vi "Andor_iXon_Point-mode.vi"(8 "Input Cluster 2":T6, 9 "Enum":enum32{"Picture", "Int Trace", "Video"}(ring), 10 "Cluster":T7) -> (0 "Output Cluster":T6, 1 "Numeric":dbl)   [LabVIEW 2009]
uses:
  atmcd32d.llb/AcquisitionMode_mode typedef.ctl
  atmcd32d.llb/ReadMode_mode typedef.ctl
  atmcd32d.llb/TriggerMode_mode typedef.ctl
  atmcd32d.llb/Shutter_type typedef.ctl
  atmcd32d.llb/Shutter_mode typedef.ctl
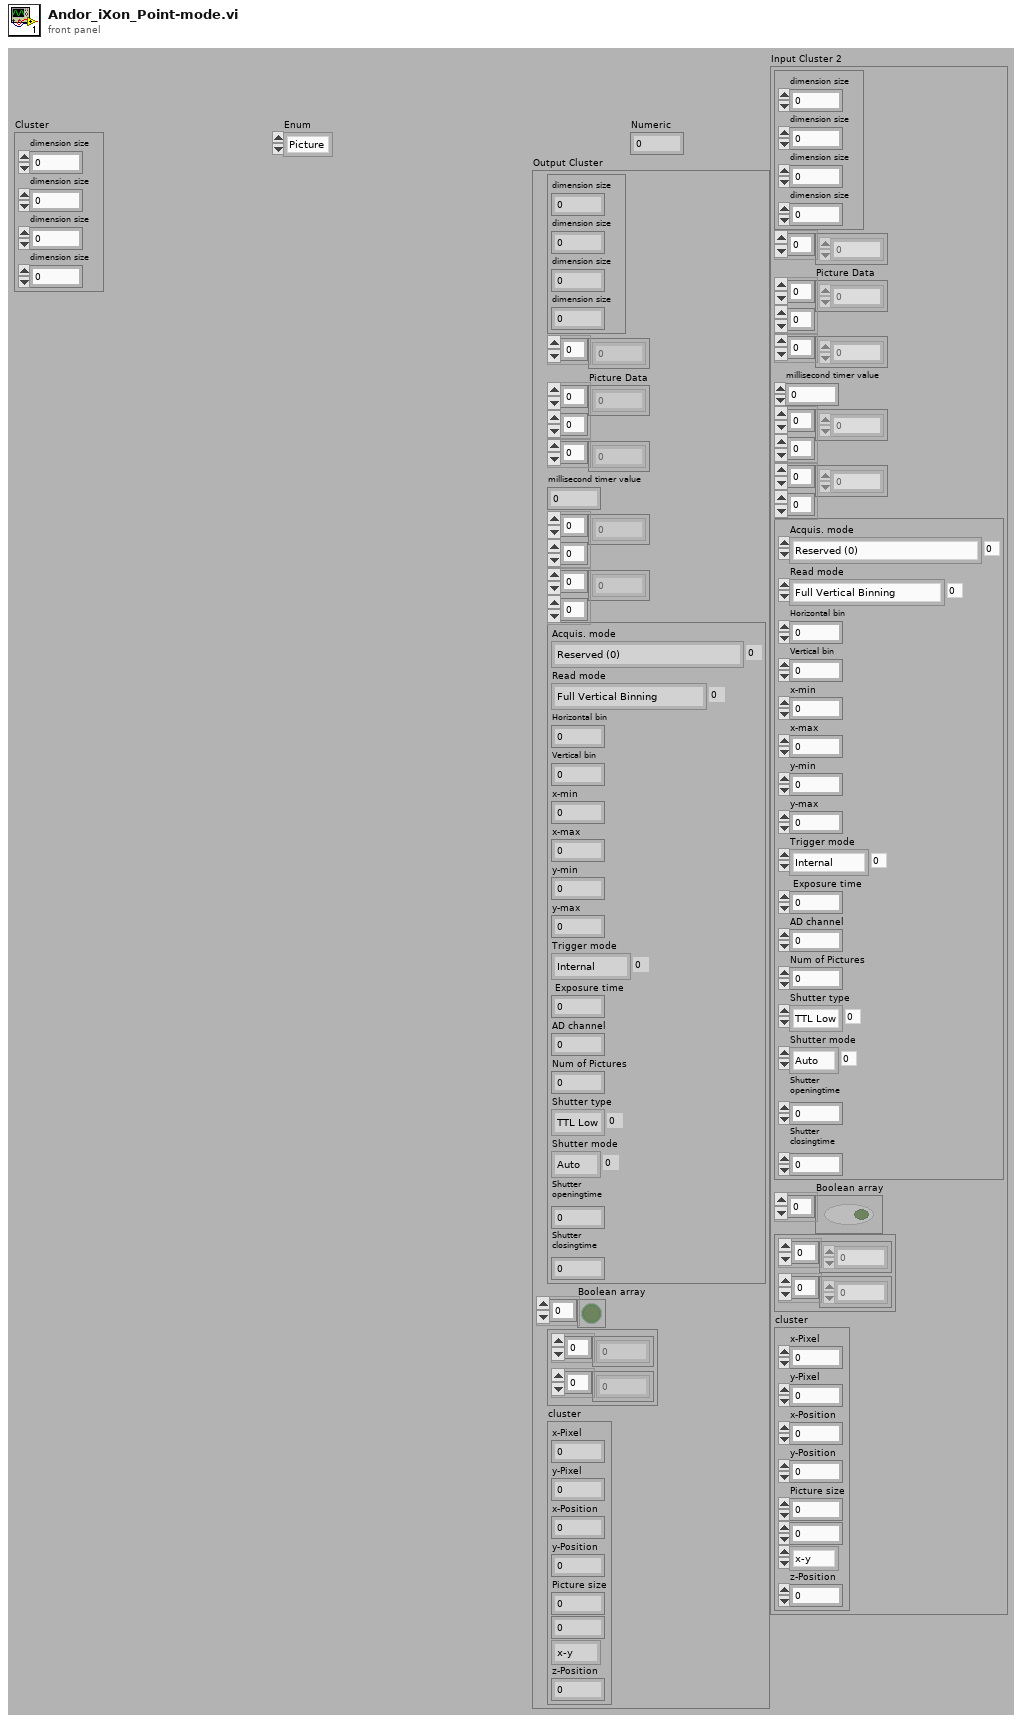
[diagram p1: front panel]
types:
  T1 = typedef "AcquisitionMode_mode typedef.ctl" = enum16{"Reserved (0)", "Single Scan", "Accumulate", "Kinetics", "Fast Kinetics", "Run Till Abort", "Reserved (6)", "Reserved (7)", "Reserved (8)", "Time Delayed Integration"}
  T2 = typedef "ReadMode_mode typedef.ctl" = enum16{"Full Vertical Binning", "Multi-Track", "Random-Track", "Single-Track", "Image"}
  T3 = typedef "TriggerMode_mode typedef.ctl" = enum16{"Internal", "External", "N/A (2)", "N/A (3)", "N/A (4)", "N/A (5)", "External Start"}
  T4 = typedef "Shutter_type typedef.ctl" = enum16{"TTL Low", "TTL High"}
  T5 = typedef "Shutter_mode typedef.ctl" = enum16{"Auto", "Open", "Close"}
  T6 = cluster{cluster{"dimension size":i32, "dimension size":i32, "dimension size":i32, "dimension size":i32}, i32[], "Picture Data":dbl[][], u32[], "millisecond timer value":u32, dbl[][], i32[][], cluster{"Acquis. mode":T1, "Read mode":T2, "Horizontal bin":i32, "Vertical bin":i32, "x-min":i32, "x-max":i32, "y-min":i32, "y-max":i32, "Trigger mode":T3, " Exposure time":sgl, "AD channel":i32, "Num of Pictures":i32, "Shutter type":T4, "Shutter mode":T5, "Shutter\nopeningtime":i32, "Shutter\nclosingtime":i32}, "Boolean array":bool[], cluster{dbl[], dbl[]}, "cluster":cluster{"x-Pixel":u16, "y-Pixel":u16, "x-Position":dbl, "y-Position":dbl, "Picture size":dbl, dbl, enum32{"x-y", "x-z", "y-z"}, "z-Position":dbl}}
  T7 = cluster{"dimension size":i32, "dimension size":i32, "dimension size":i32, "dimension size":i32}
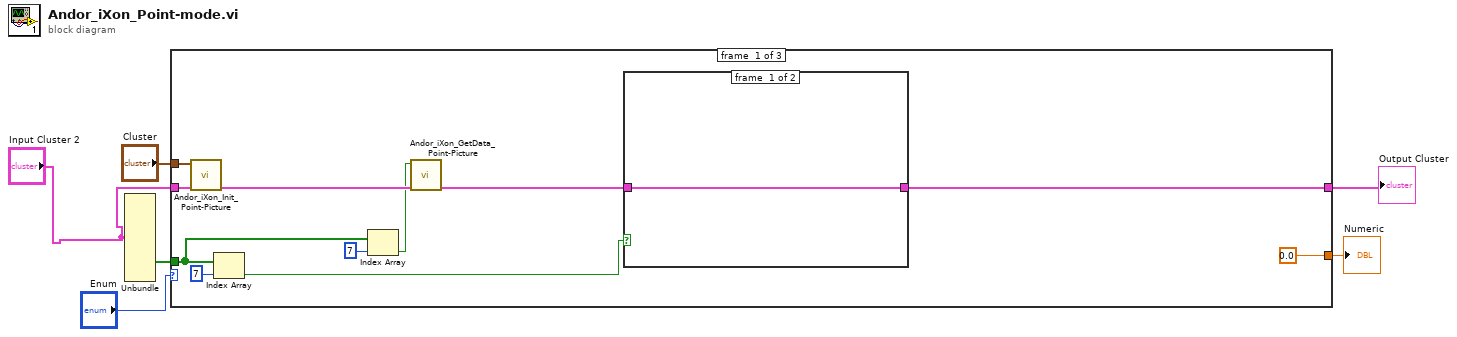
[diagram p0: block diagram]
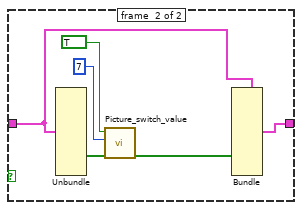
[diagram p2: hidden frame]
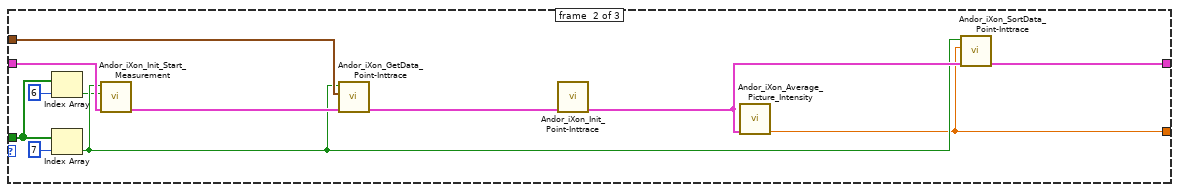
[diagram p3: hidden frame]
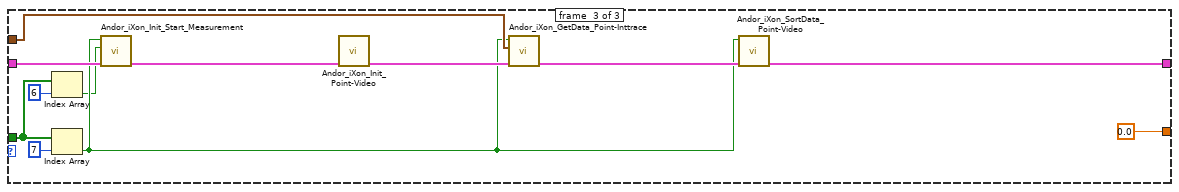
[diagram p4: hidden frame]
diagram:
  n1 = Unbundle("Input Cluster 2") -> ("Boolean array"=w3:bool[])  [unwired: 10 out]
  n2 = case shown="\"Video\"" "Enum" {
    tunnel: [w17 w32 w44] -> w2
    tunnel: "Cluster" -> [w13 w35 w47]
    tunnel: "Input Cluster 2" -> [w8 w31 w43]
    tunnel: w3 -> [w15 w27 w39]
    tunnel: [0.0 ("Numeric") w25 0.0 ("Numeric")] -> w5
    frame #0 {
      n3 = call "Andor_iXon_Init_Point-Picture.vi"("Input Cluster 2"=w8, "Cluster"=w13) -> ("Output Cluster"=w14:T6)  [unwired: 9 out]
      n4 = Index Array(array=w15, index=7) -> (element=w9:bool)
      n5 = Index Array(array=w15, index=7) -> (element=w11:bool)
      n6 = call "Andor_iXon_GetData_Point-Picture.vi"("Input Cluster"=w14, "Measure"=w11) -> ("Output Cluster"=w16:T6)  [unwired: 9 out]
      n7 = case shown="True" w9 {
        tunnel: w16 -> [w18 w21]
        tunnel: [w18 w19] -> w17
        frame #0 {
        }
        frame #1 {
          n8 = Unbundle(w21) -> ("Boolean array"=w22:bool[])  [unwired: 10 out]
          n9 = call "Picture_switch_value.vi"("Boolean array in"=w22, "Value to switch"=7, "Switch"=TRUE) -> ("Boolean array out"=w20:bool[])  [unwired: 8 out]
          n10 = Bundle(cluster=w21, "Boolean array"=w20) -> (w19:T6)  [unwired: 10 out]
        }
      }
    }
    frame #1 {
      n11 = Index Array(array=w27, index=6) -> (element=w26:bool)
      n12 = Index Array(array=w27, index=7) -> (element=w29:bool)
      n13 = call "Andor_iXon_Init_Start_Measurement.vi"("Input Cluster 2"=w31, "change"=w26, "Init"=w29) -> ("Input Cluster 3"=w30:T6)  [unwired: 8 out]
      n14 = call "Andor_iXon_GetData_Point-Inttrace.vi"("Input Cluster"=w30, "Cluster"=w35, "Measure"=w29) -> ("Output Cluster"=w34:T6)  [unwired: 8 out]
      n15 = call "Andor_iXon_Init_Point-Inttrace.vi"("Input Cluster"=w34) -> ("Input Cluster 2"=w33:T6)  [unwired: 10 out]
      n16 = call "Andor_iXon_Average_Picture_Intensity.vi"("Input Cluster"=w33) -> ("Numeric"=w25:dbl)  [unwired: 10 out]
      n17 = call "Andor_iXon_SortData_Point-Inttrace.vi"("Input Cluster"=w33, "Numeric"=w25, "Boolean"=w29) -> ("Output Cluster"=w32:T6)  [unwired: 8 out]
    }
    frame #2 {
      n18 = Index Array(array=w39, index=6) -> (element=w38:bool)
      n19 = Index Array(array=w39, index=7) -> (element=w41:bool)
      n20 = call "Andor_iXon_Init_Start_Measurement.vi"("Input Cluster 2"=w43, "change"=w38, "Init"=w41) -> ("Input Cluster 3"=w42:T6)  [unwired: 8 out]
      n21 = call "Andor_iXon_Init_Point-Video.vi"("Input Cluster"=w42) -> ("output cluster"=w46:T6)  [unwired: 10 out]
      n22 = call "Andor_iXon_GetData_Point-Inttrace.vi"("Input Cluster"=w46, "Cluster"=w47, "Measure"=w41) -> ("Output Cluster"=w45:T6)  [unwired: 8 out]
      n23 = call "Andor_iXon_SortData_Point-Video.vi"("Input Cluster"=w45, "Sort"=w41) -> ("Output Cluster"=w44:T6)  [unwired: 9 out]
    }
  }
  "Numeric" <- w5
  "Output Cluster" <- w2
